vi "9478_UI.vi"(8 "error in (no error)":errorcluster, 11 "Node Ptr":T2 format="%.0x") -> (0 "error out":errorcluster)   [LabVIEW 2017, in "Modules.lvlib" / "9478.lvclass"]
uses:
  9478.lvclass
  <vilib>/NI Veristand/Custom Device API/Custom Device Item Ref.ctl
  RSI Module/SubPanel Command.ctl
  Active Limit.ctl
  C:/Users/dbuck/Documents/GitHub/Scan-Engine-Custom-Device-Classes/Source/RSI Module/RSI Module.lvclass
  9478.lvclass/9478.ctl
  RSI Module/RSI Module.lvclass
  <vilib>/NI Veristand/Custom Device API/Custom Device API.lvlib
panel:
  in  "_UpdateModSettings":bool
  out "_Active Limit Label":string="Active Limits"
  out "_Module Settings Label":string="Module Settings"
  out "_Selected Channel(s) Settings Label":string="Selected Channel(s) Settings"
  out "_Amps Label 2":string="Amps"
  out "_Amps Label":string="Amps"
  out "_US Label":string="us"
  in  "Overcurrent Refresh\nPeriod":dbl=20.0 min=20.0 max=2550.0 step=10.0
  in  "Enable Overcurrent \nRefresh":bool
  in  "Current Limit B":dbl=1.2000000476837158 min=0.0 max=5.099999904632568 step=0.019999999552965164
  in  "Current Limit A":dbl=1.2000000476837158 min=0.0 max=5.099999904632568 step=0.019999999552965164
  in  "Bad Active Limit":u8(ring) items=["Limit A"=1, "Limit B"=2, "No Limit"=3, "X"=4]
  in  "Active Limit":T1=1 items=["Limit A"=1, "Limit B"=2, "No Limit"=3]
  in  "Channels":i32[](listbox)=[0]
  in  "SubPanel Event":refnum<user-event>
  in  "Header":cluster{"Section Name":string}={"Section Name"="NI 9205 Settings"}
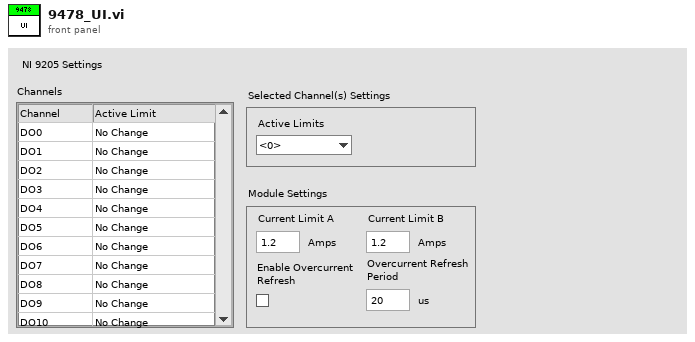
[diagram p1: front panel]
types:
  T1 = typedef "Modules.lvlib/9478.lvclass/Active Limit.ctl" = u8
  T2 = typedef "Custom Device API.lvlib/Custom Device Item Ref.ctl" = u64
  T3 = typedef "Modules.lvlib/RSI Module.lvclass/Module Models.ctl" = enum16{"Empty", "NI 9201", "NI 9203", "NI 9205", "NI 9206", "NI 9207", "NI 9208", "NI 9211", "NI 9212", "NI 9213", "NI 9214", "NI 9215", "NI 9217", "NI 9219", "NI 9220", "NI 9221", "NI 9222", "NI 9223", "NI 9225", "NI 9227", "NI 9229", "NI 9233", "NI 9234", "NI 9235", "NI 9236", "NI 9237", "NI 9239", "NI 9242", "NI 9244", "NI 9263", "NI 9264", "NI 9265", "NI 9269", "NI 9375", "NI 9401", "NI 9402", "NI 9403", "NI 9411", "NI 9421", "NI 9422", "NI 9423", "NI 9425", "NI 9426", "NI 9435", "NI 9437", "NI 9472", "NI 9474", "NI 9475", "NI 9476", "NI 9477", "NI 9478", "NI 9481", "NI 9482", "NI 9485"}
  T4 = typedef "Modules.lvlib/RSI Module.lvclass/SubPanel Command.ctl" = enum16{"Stop"}
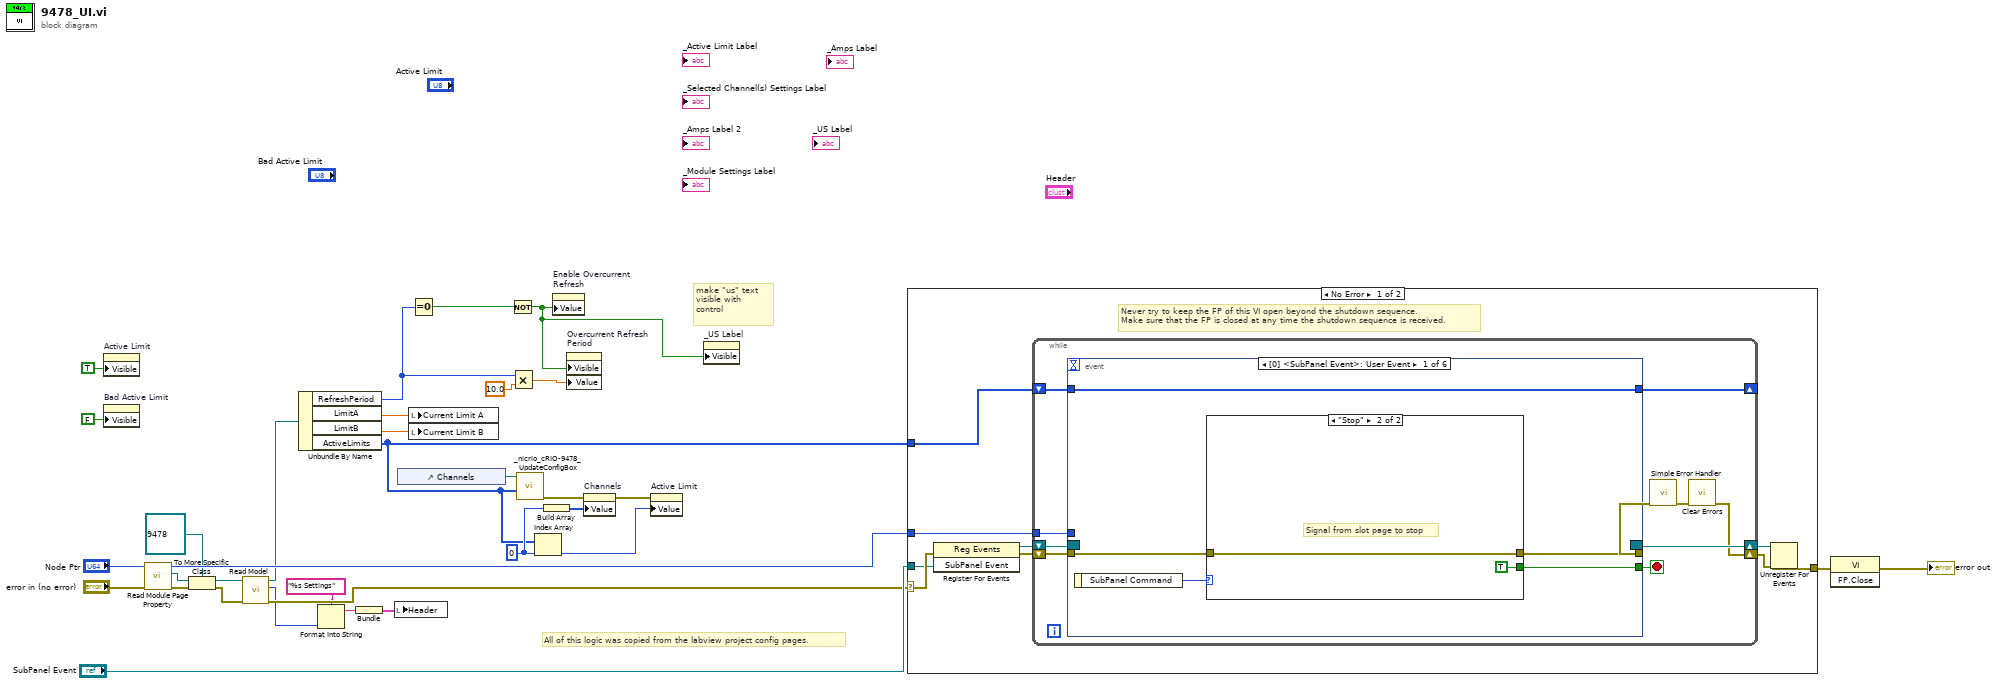
[diagram p0: block diagram]
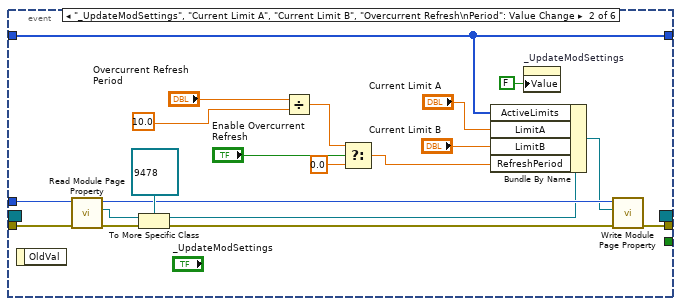
[diagram p3: hidden frame]
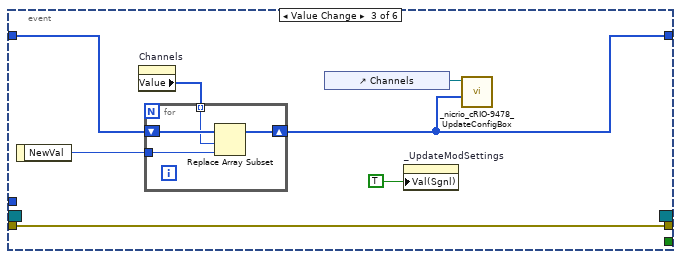
[diagram p4: hidden frame]
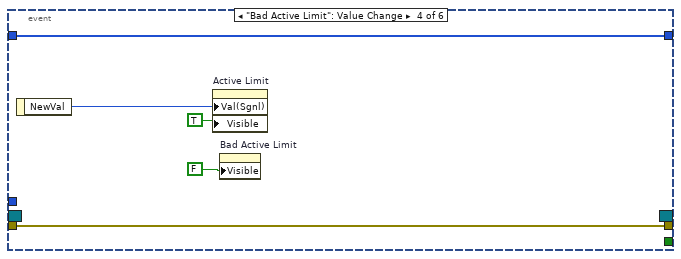
[diagram p5: hidden frame]
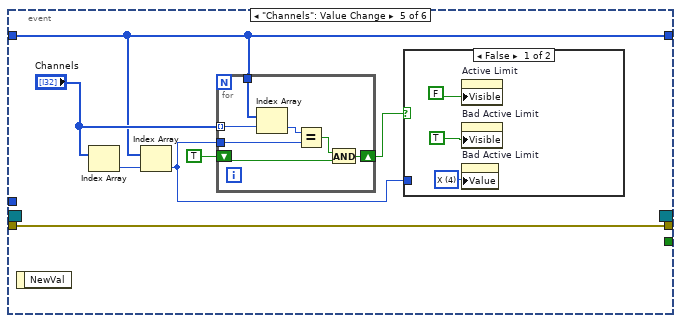
[diagram p6: hidden frame]
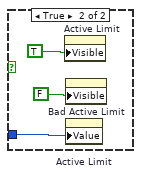
[diagram p7: hidden frame]
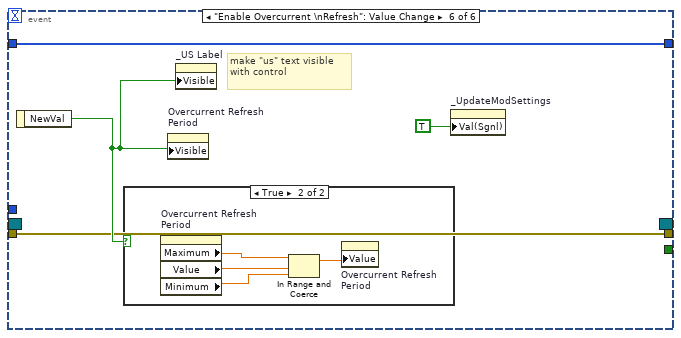
[diagram p8: hidden frame]
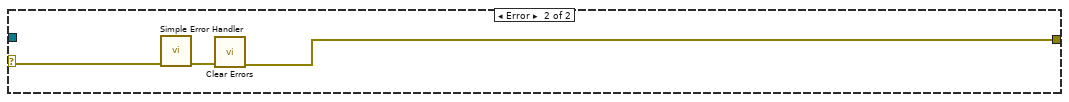
[diagram p10: hidden frame]
diagram:
  w3 = 0 ("index")
  # "All of this logic was copied from the labview project config pages."
  # "make \"us\" text visible with control"
  n1 = property on="Active Limit" class="Ring (strict)"("Visible"=TRUE) -> ()  [unwired: 2 in, 2 out]
  n2 = property on="Bad Active Limit" class="Ring (strict)"("Visible"=FALSE) -> ()  [unwired: 2 in, 2 out]
  n3 = call "Read Module Page Property.vi"("error in (no error)"="error in (no error)", "Node Ptr In"="Node Ptr") -> ("error out"=w24:errorcluster, "RSI Module"=w22:refnum<class "RSI Module.lvclass">, "Node Ptr Out"=w30:T2)  [unwired: 7 in]
  n4 = To More Specific Class(target class=refnum<class "9478.lvclass"> refnum ("9205 in"), reference=w22, error in=w24) -> (specific class reference=w21:refnum<class "9478.lvclass">, error out=w20:errorcluster)
  n5 = call "Read Model.vi"("error in (no error)"=w20, "RSI Module in"=w21) -> ("error out"=w27:errorcluster, "Model"=w18:T3, "RSI Module out"=w15:refnum<class "9478.lvclass">)  [unwired: 7 in]
  n6 = Unbundle By Name(w15) -> ("RefreshPeriod"=w8:u8, "LimitA"=w14:dbl, "LimitB"=w13:dbl, "ActiveLimits"=w1:T1[])
  n7 = Format Into String(format string="%s Settings", w18) -> (resulting string=w16:string)  [unwired: 2 in, 1 out]
  n8 = Bundle(w16) -> (w19:cluster{string})  [unwired: 1 in]
  n9 = local write "Header"(w19) -> ()
  n10 = control-ref of="Channels"() -> (w7:refnum<vi>)
  n11 = local write "Current Limit A"(w14) -> ()
  n12 = local write "Current Limit B"(w13) -> ()
  n13 = Equal To 0?(x=w8) -> (x = 0?=w10:bool)
  n14 = Not(x=w10) -> (.not. x?=w12:bool)
  n15 = Multiply(x=w8, y=10.0) -> (x*y=w11:dbl)
  n16 = call "_nicrio_cRIO-9478_UpdateConfigBox.vi"("Active Limit"=w1, "Channel Refnum"=w7) -> ("error out"=w2:errorcluster)  [unwired: 8 in, 1 out]
  n17 = Index Array(array=w1, index=w3) -> (element=w6:T1)
  n18 = Build Array(w3) -> (w4:i32[])
  n19 = property on="Enable Overcurrent \nRefresh" class="Bool (strict)"("Value"=w12) -> ()  [unwired: 2 in, 2 out]
  n20 = property on="Overcurrent Refresh\nPeriod" class="DigNum (strict)"("Visible"=w12, "Value"=w11) -> ()  [unwired: 2 in, 2 out]
  n21 = property on="Channels" class="MCListbox (strict)"(error in=w2, "Value"=w4) -> (error out=w5:errorcluster)  [unwired: 1 in, 1 out]
  n22 = property on="Active Limit" class="Ring (strict)"(error in=w5, "Value"=w6) -> ()  [unwired: 1 in, 2 out]
  n23 = property on="_US Label" class="Str"("Visible"=w12) -> ()  [unwired: 2 in, 2 out]
  n24 = case shown="No Error" w27 {
    selector: w27 -> [w36 w127]
    tunnel: [w40 w125] -> w33
    tunnel: w30 -> [w37 _]
    tunnel: "SubPanel Event" -> [w35 _]
    tunnel: w1 -> [w34 _]
    frame No Error {
      # "Never try to keep the FP of this VI open beyond the shutdown sequence.\nMake sure that the FP is closed at any time the shutdown sequence is received."
      n25 = register-events(error in=w36, w35) -> (reference out=w38:refnum<event-registration>, error out=w39:errorcluster)  [unwired: 1 in]
      n26 = while {
        tunnel: w37 -> [w48]
        shift-right: [w45] -> w41
        shift-left: w39 -> [w51]
        shift-right: [w52] -> w42
        shift-left: w38 -> [w50]
        shift-right: [w44] -> _
        shift-left: w34 -> [w43]
        stop <- w49 stop-if-true
        n27 = event shown="[0] <SubPanel Event>: User Event" {
          selector: w50 -> [_ _ _ _ _ _]
          dyn-events: [_ _ _ _ _ _] -> w52
          timeout: _ -> [_ _ _ _ _ _]
          tunnel: w51 -> [w56 w74 w82 w93 w97 w118]
          tunnel: [w55 _ _ _ _ _] -> w49
          tunnel: [w54 w73 w82 w93 w97 w118] -> w47
          tunnel: w48 -> [_ w75 _ _ _ _]
          tunnel: [w53 w69 w83 w96 w98 w120] -> w44
          tunnel: w43 -> [w53 w69 w86 w96 w98 w120]
          event User Event {
            n28 = event-data() -> ("SubPanel Command"=w57:T4)  [unwired: 1 out]
            n29 = case shown="\"Stop\"" w57 {
              tunnel: w56 -> [w58 w59]
              tunnel: [w58 w59] -> w54
              tunnel: [_ TRUE] -> w55
              frame Default {
              }
              frame "Stop" {
                # "Signal from slot page to stop"
              }
            }
          }
          event "_UpdateModSettings", "Current Limit A", "Current Limit B", "Overcurrent Refresh\nPeriod": Value Change {
            n30 = event-data() -> ()  [unwired: 2 out]
            n31 = call "Read Module Page Property.vi"("error in (no error)"=w74, "Node Ptr In"=w75) -> ("error out"=w78:errorcluster, "RSI Module"=w79:refnum<class "RSI Module.lvclass">, "Node Ptr Out"=w76:T2)  [unwired: 7 in]
            n32 = To More Specific Class(target class=refnum<class "9478.lvclass"> refnum ("9205 in"), reference=w79, error in=w78) -> (specific class reference=w72:refnum<class "9478.lvclass">, error out=w77:errorcluster)
            n33 = Divide(x="Overcurrent Refresh\nPeriod", y=10.0 ("f")) -> (x/y=w65:dbl)
            n34 = Select(t=w65, s="Enable Overcurrent \nRefresh", f=0.0) -> (s? t:f=w62:dbl)
            n35 = Bundle By Name(cluster=w72, "ActiveLimits"=w69, "LimitA"="Current Limit A", "LimitB"="Current Limit B", "RefreshPeriod"=w62) -> (w71:refnum<class "9478.lvclass">)
            n36 = property on="_UpdateModSettings" class="Bool (strict)"("Value"=FALSE ("_UpdateModSettings")) -> ()  [unwired: 2 in, 2 out]
            n37 = call "Write Module Page Property.vi"("error in (no error)"=w77, "RSI Module"=w71, "Node Ptr In"=w76) -> ("error out"=w73:errorcluster)  [unwired: 6 in, 2 out]
          }
          event Value Change {
            n38 = event-data() -> ("NewVal"=w85:T1)  [unwired: 1 out]
            n39 = property on="Channels" class="MCListbox (strict)"() -> ("Value"=w87:i32[])  [unwired: 2 in, 2 out]
            n40 = for {
              tunnel: w85 -> [w89]
              tunnel: w87 -> [w88] mode=indexing
              shift-right: [w91] -> w83
              shift-left: w86 -> [w90]
              n41 = Replace Array Subset(array=w90, new element=w89, index=w88) -> (w91:T1[])
            }
            n42 = control-ref of="Channels"() -> (w84:refnum<vi>)
            n43 = property on="_UpdateModSettings" class="Bool (strict)"("Val(Sgnl)"=TRUE ("_UpdateModSettings")) -> ()  [unwired: 2 in, 2 out]
            n44 = call "_nicrio_cRIO-9478_UpdateConfigBox.vi"("Active Limit"=w83, "Channel Refnum"=w84) -> ()  [unwired: 8 in, 2 out]
          }
          event "Bad Active Limit": Value Change {
            n45 = event-data() -> ("NewVal"=w92:u8)  [unwired: 1 out]
            n46 = property on="Active Limit" class="Ring (strict)"("Val(Sgnl)"=w92, "Visible"=TRUE) -> ()  [unwired: 2 in, 2 out]
            n47 = property on="Bad Active Limit" class="Ring (strict)"("Visible"=FALSE) -> ()  [unwired: 2 in, 2 out]
          }
          event "Channels": Value Change {
            n48 = event-data() -> ()  [unwired: 2 out]
            n49 = Index Array(array="Channels") -> (element=w101:i32)  [unwired: 1 in]
            n50 = Index Array(array=w98, index=w101) -> (element=w103:T1)
            n51 = for {
              tunnel: "Channels" -> [w115] mode=indexing
              tunnel: w98 -> [w116]
              tunnel: w103 -> [w113]
              shift-right: [w111] -> w102
              shift-left: TRUE -> [w110]
              n52 = Index Array(array=w116, index=w115) -> (element=w114:T1)
              n53 = Equal?(x=w114, y=w113) -> (x = y?=w112:bool)
              n54 = And(x=w112, y=w110) -> (x .and. y?=w111:bool)
            }
            n55 = case shown="False" w102 {
              tunnel: w103 -> [_ w108]
              frame False {
                w104 = u8 4 items=["Limit A"=1, "Limit B"=2, "No Limit"=3, "X"=4] ("Bad Active Limit")
                n56 = property on="Active Limit" class="Ring (strict)"("Visible"=FALSE) -> ()  [unwired: 2 in, 2 out]
                n57 = property on="Bad Active Limit" class="Ring (strict)"("Visible"=TRUE) -> ()  [unwired: 2 in, 2 out]
                n58 = property on="Bad Active Limit" class="Ring (strict)"("Value"=w104) -> ()  [unwired: 2 in, 2 out]
              }
              frame True {
                n59 = property on="Active Limit" class="Ring (strict)"("Visible"=TRUE) -> ()  [unwired: 2 in, 2 out]
                n60 = property on="Bad Active Limit" class="Ring (strict)"("Visible"=FALSE) -> ()  [unwired: 2 in, 2 out]
                n61 = property on="Active Limit" class="Ring (strict)"("Value"=w108) -> ()  [unwired: 2 in, 2 out]
              }
            }
          }
          event "Enable Overcurrent \nRefresh": Value Change {
            # "make \"us\" text visible with control"
            n62 = event-data() -> ("NewVal"=w119:bool)  [unwired: 1 out]
            n63 = case shown="True" w119 {
              frame False {
              }
              frame True {
                n64 = property on="Overcurrent Refresh\nPeriod" class="DigNum (strict)"() -> ("Maximum"=w123:dbl, "Value"=w122:dbl, "Minimum"=w121:dbl)  [unwired: 2 in, 2 out]
                n65 = In Range and Coerce(upper limit=w123, x=w122, lower limit=w121) -> (coerced(x)=w124:dbl)  [unwired: 1 out]
                n66 = property on="Overcurrent Refresh\nPeriod" class="DigNum (strict)"("Value"=w124) -> ()  [unwired: 2 in, 2 out]
              }
            }
            n67 = property on="Overcurrent Refresh\nPeriod" class="DigNum (strict)"("Visible"=w119) -> ()  [unwired: 2 in, 2 out]
            n68 = property on="_US Label" class="Str"("Visible"=w119) -> ()  [unwired: 2 in, 2 out]
            n69 = property on="_UpdateModSettings" class="Bool (strict)"("Val(Sgnl)"=TRUE ("_UpdateModSettings")) -> ()  [unwired: 2 in, 2 out]
          }
        }
        n70 = call <vilib>:"Simple Error Handler.vi"("error in (no error)"=w47) -> ("error out"=w46:errorcluster)  [unwired: 1 in, 7 out]
        n71 = call <vilib>:"Clear Errors.vi"("error in (no error)"=w46) -> ("error out"=w45:errorcluster)  [unwired: 1 in, 5 out]
      }
      n72 = Unregister For Events(event registration refnum=w42, error in=w41) -> (error out=w40:errorcluster)
    }
    frame Error {
      n73 = call <vilib>:"Simple Error Handler.vi"("error in (no error)"=w127) -> ("error out"=w126:errorcluster)  [unwired: 1 in, 7 out]
      n74 = call <vilib>:"Clear Errors.vi"("error in (no error)"=w126) -> ("error out"=w125:errorcluster)  [unwired: 1 in, 5 out]
    }
  }
  n75 = invoke class="VI" method="FP.Close"(error in=w33) -> (error out=→"error out":errorcluster)  [unwired: 2 in, 2 out]
